vi "move-targer-eventSD.vi"(0 "cellule":u16(ring)=1 items=["Cellule 1 circulation", "Cellule statique", "Lanex", "Cellule 2 circulation"], 1 "NewVal":variant, 2 "reference in":refnum<vi>, 3 "pos of targets":dbl[](array[numeric])=[15.8, 0.0, -12.0, -23.0]) -> ()   [LabVIEW 2015]
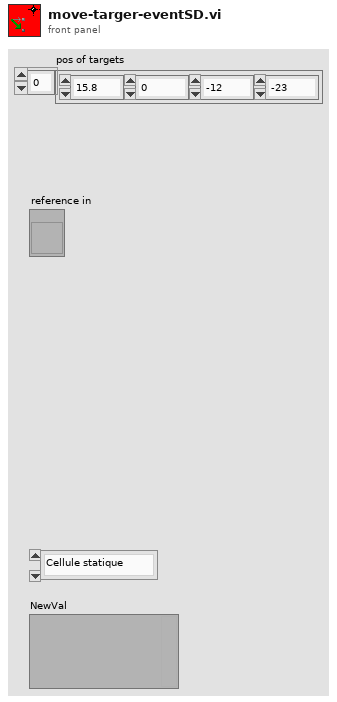
[diagram p1: front panel]
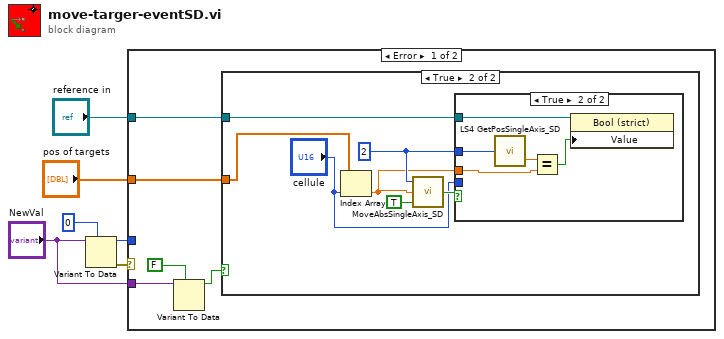
[diagram p0: block diagram]
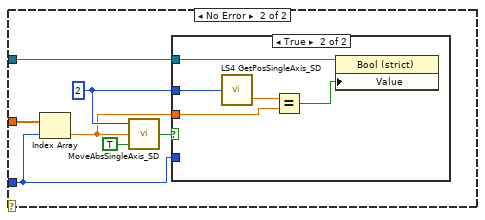
[diagram p4: hidden frame]
diagram:
  n1 = Variant To Data(type=0, Variant="NewVal") -> (data=w6:i32, error out=w5:errorcluster)  [unwired: 1 in]
  n2 = case shown="Error" w5 {
    tunnel: "NewVal" -> [w11 _]
    tunnel: w6 -> [_ w25]
    tunnel: "reference in" -> [w8 w27]
    tunnel: "pos of targets" -> [w7 w26]
    frame Error {
      n3 = Variant To Data(type=FALSE, Variant=w11) -> (data=w9:bool)  [unwired: 1 in, 1 out]
      n4 = case shown="True" w9 {
        tunnel: w8 -> [_ w15]
        tunnel: w7 -> [_ w14]
        frame False {
        }
        frame True {
          w18 = 2 ("Axis")
          n5 = Index Array(array=w14, index="cellule") -> (element=w12:dbl)
          n6 = call "MoveAbsSingleAxis_SD.vi"("Wait"=TRUE, "Value"=w12, "Axis"=w18) -> ("Command executed"=w17:bool)
          n7 = case shown="True" w17 {
            tunnel: w18 -> [_ w22]
            tunnel: "cellule" -> [_ _]
            tunnel: w15 -> [_ w20]
            tunnel: w12 -> [_ w19]
            frame False {
            }
            frame True {
              n8 = call "LS4 GetPosSingleAxis_SD.vi"("Axis"=w22) -> ("Pos"=w23:dbl)  [unwired: 1 out]
              n9 = Equal?(x=w23, y=w19) -> (x = y?=w21:bool)
              n10 = property class="Bool (strict)"(reference=w20, "Value"=w21) -> ()  [unwired: 1 in, 2 out]
            }
          }
        }
      }
    }
    frame No Error {
      w30 = 2 ("Axis")
      n11 = Index Array(array=w26, index=w25) -> (element=w24:dbl)
      n12 = call "MoveAbsSingleAxis_SD.vi"("Wait"=TRUE, "Value"=w24, "Axis"=w30) -> ("Command executed"=w29:bool)
      n13 = case shown="True" w29 {
        tunnel: w30 -> [_ w34]
        tunnel: w25 -> [_ _]
        tunnel: w27 -> [_ w32]
        tunnel: w24 -> [_ w31]
        frame False {
        }
        frame True {
          n14 = call "LS4 GetPosSingleAxis_SD.vi"("Axis"=w34) -> ("Pos"=w35:dbl)  [unwired: 1 out]
          n15 = Equal?(x=w35, y=w31) -> (x = y?=w33:bool)
          n16 = property class="Bool (strict)"(reference=w32, "Value"=w33) -> ()  [unwired: 1 in, 2 out]
        }
      }
    }
  }
